vi "Path selector.vi"(8 "error in (no error)":errorcluster, 11 "start path (directory)":path=path "C:/Users/user/Documents/LabVIEW Data/data" caption="start path") -> (0 "error out":errorcluster, 3 "selected path (directory)":path caption="selected path")   [LabVIEW 2020]
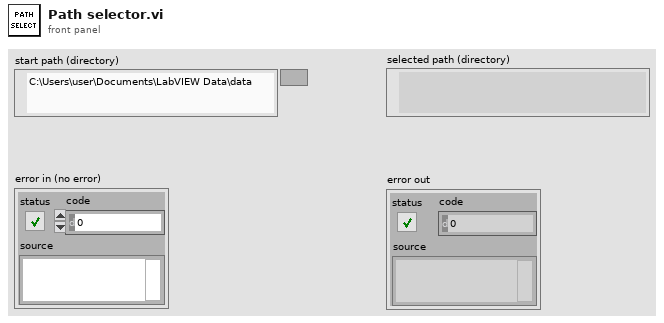
[diagram p1: front panel]
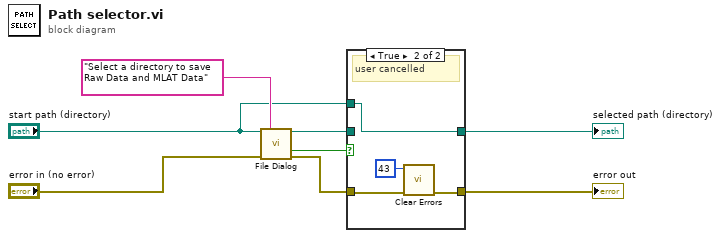
[diagram p0: block diagram]
diagram:
  n1 = call "File Dialog"("start path"="start path (directory)", "prompt"="Select a directory to save Raw Data and MLAT Data", "error in"="error in (no error)") -> ("selected path"=w4:path, "cancelled"=w6:bool, "error out"=w5:errorcluster)  [unwired: 9 in, 1 out]
  n2 = case shown="True" w6 {
    tunnel: w5 -> [w9 w13]
    tunnel: w4 -> [w10 _]
    tunnel: "start path (directory)" -> [_ w14]
    tunnel: [w10 w14] -> w2
    tunnel: [w9 w12] -> w1
    frame False {
    }
    frame True {
      # "user cancelled"
      n3 = call <vilib>:"Clear Errors.vi"("error in (no error)"=w13, "specific error code to clear (0: all)"=43) -> ("error out"=w12:errorcluster)  [unwired: 4 in, 1 out]
    }
  }
  "selected path (directory)" <- w2
  "error out" <- w1
